vi "stats.vi"(2 "ArrayIn":dbl[](array[numeric])) -> (7 "stats":dbl[](array[numeric]))   [LabVIEW 2014]
uses:
  <vilib>/Analysis/NI_AALBase.lvlib
  <vilib>/gmath/NI_Gmath.lvlib
panel:
  in  "cdf(x)":dbl=0.025
  # "(1 - probability) / 2"
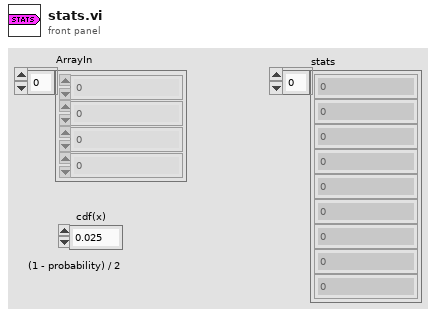
[diagram p1: front panel]
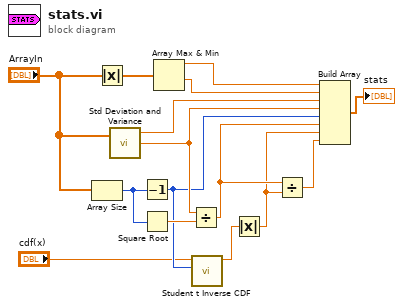
[diagram p0: block diagram]
diagram:
  n1 = Array Size(array="ArrayIn") -> (size(s)=w9:i32)
  n2 = Absolute Value(x="ArrayIn") -> (abs(x)=w11:dbl[])
  n3 = call <vilib>:"Std Deviation and Variance.vi"("X"="ArrayIn") -> ("mean"=w15:dbl, "standard deviation"=w7:dbl)  [unwired: 1 in, 1 out]
  n4 = Decrement(x=w9) -> (x-1=w6:i32)
  n5 = Square Root(x=w9) -> (sqrt(x)=w8:dbl)
  n6 = Array Max & Min(array=w11) -> (max value=w13:dbl, min value=w12:dbl)  [unwired: 2 out]
  n7 = Divide(x=w7, y=w8) -> (x/y=w3:dbl)
  n8 = call <vilib>:"Student t Inverse CDF.vi"("k degrees of freedom"=w6, "cdf(x)"="cdf(x)") -> ("x"=w4:dbl)  [unwired: 8 in, 1 out]
  n9 = Absolute Value(x=w4) -> (abs(x)=w2:dbl)
  n10 = Divide(x=w3, y=w2) -> (x/y=w1:dbl)
  n11 = Build Array(w13, w12, w15, w7, w6, w3, w2, w1) -> (→"stats":dbl[])
